vi "DE_Get Best Min.vi"(8 "error in (no error)":errorcluster, 9 "State In":T1) -> (0 "error out":errorcluster, 1 "State Out":T1, 2 "F(Minimum)":dbl[](array[numeric]), 3 "Minimum":dbl[](array[numeric]))   [LabVIEW 2020, in "NI_AAL_GlobalOptimization.lvlib"]
uses:
  <vilib>/gmath/NI_AAL_GlobalOptimization.lvlib
  <vilib>/gmath/GlobalOptimization.llb/DE_State.ctl
  <vilib>/gmath/GlobalOptimization.llb/DE_Population.ctl
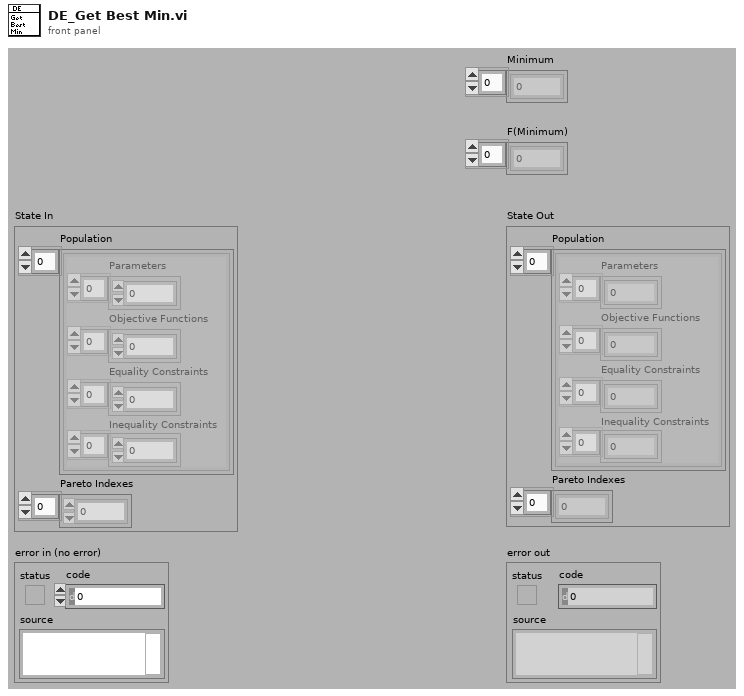
[diagram p1: front panel]
types:
  T1 = typedef "NI_AAL_GlobalOptimization.lvlib/DE_State.ctl" = cluster{"Population":T2[], "Pareto Indexes":i32[]}
  T2 = typedef "NI_AAL_GlobalOptimization.lvlib/DE_Population.ctl" = cluster{"Parameters":dbl[], "Objective Functions":dbl[], "Equality Constraints":dbl[], "Inequality Constraints":dbl[]}
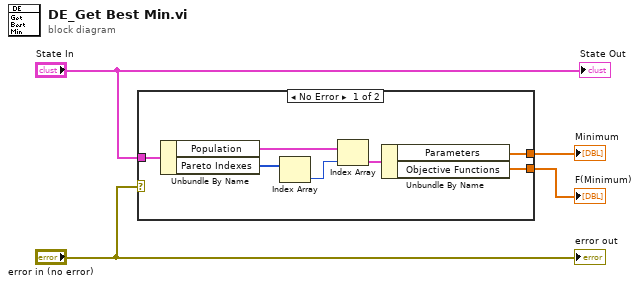
[diagram p0: block diagram]
diagram:
  n1 = case shown="No Error" "error in (no error)" {
    tunnel: "State In" -> [w7 _]
    tunnel: [w6 _] -> w4
    tunnel: [w5 _] -> w3
    frame No Error {
      n2 = Unbundle By Name(w7) -> ("Population"=w10:T2[], "Pareto Indexes"=w11:i32[])
      n3 = Index Array(array=w11) -> (element=w9:i32)  [unwired: 1 in]
      n4 = Index Array(array=w10, index=w9) -> (element=w8:T2)
      n5 = Unbundle By Name(w8) -> ("Parameters"=w6:dbl[], "Objective Functions"=w5:dbl[])
    }
    frame Error {
    }
  }
  "Minimum" <- w4
  "F(Minimum)" <- w3
  "error out" <- "error in (no error)"
  "State Out" <- "State In"
